vi "XYStage_Initialize_Ludl_Kinetec.vi"(8 "error in (no error)":errorcluster, 11 "VISA resource name":refnum<visa-resource-name>) -> (0 "error out":errorcluster, 3 "VISA resource name out":refnum<visa-resource-name>)   [LabVIEW 2013]
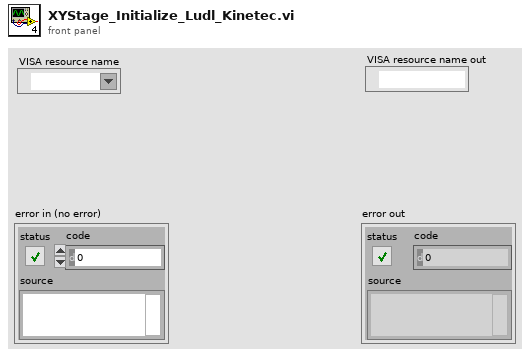
[diagram p1: front panel]
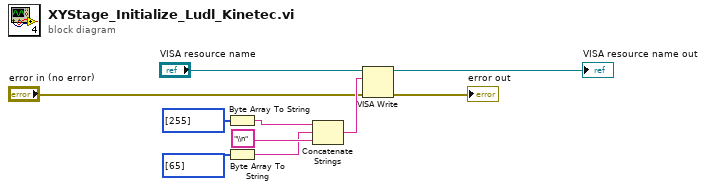
[diagram p0: block diagram]
diagram:
  n1 = Byte Array To String(unsigned byte array=u8[] [255]) -> (string=w7:string)
  n2 = Byte Array To String(unsigned byte array=u8[] [65]) -> (string=w9:string)
  n3 = Concatenate Strings(w7, w9, "\\n") -> (w5:string)
  n4 = VISA Write(VISA resource name="VISA resource name", write buffer=w5, error in (no error)="error in (no error)") -> (VISA resource name out=→"VISA resource name out":refnum<visa-resource-name>, error out=→"error out":errorcluster)  [unwired: 1 out]
